vi "api_token.read.vi"(8 "error in":errorcluster, 11 "Nominal Client in":refnum<class "Nominal Client.lvclass">) -> (0 "error out":errorcluster, 2 "API Token":string, 3 "Nominal Client out":refnum<class "Nominal Client.lvclass">)   [LabVIEW 2020, in "Nominal Client.lvclass"]
uses:
  Nominal Client.lvclass
  Nominal Client.lvclass/Nominal Client.ctl
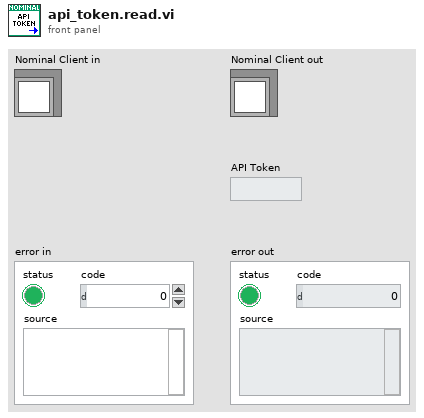
[diagram p1: front panel]
types:
  T1 = typedef "Nominal Client.lvclass/private_data.ctl" = cluster{"API Token":string, "REST Client":refnum<class "REST Client.lvclass">}
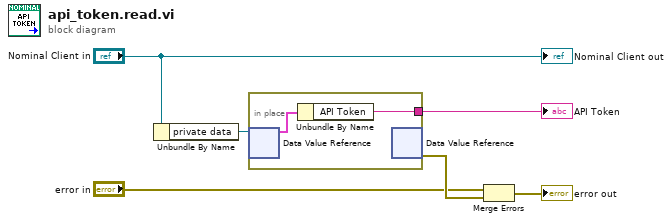
[diagram p0: block diagram]
diagram:
  n1 = Unbundle By Name("Nominal Client in") -> ("private data"=w6:refnum<data-value>)
  n2 = in-place {
    in-place-border: [w7] -> w5
    n3 = in-place-dvr #1(w6) -> (w8:T1)  [unwired: 1 out]
    n4 = Unbundle By Name(w8) -> ("API Token"=w7:string)
    n5 = in-place-dvr #1() -> (w3:errorcluster)  [unwired: 1 in, 1 out]
  }
  "API Token" <- w5
  n6 = Merge Errors("error in", w3) -> (→"error out":errorcluster)
  "Nominal Client out" <- "Nominal Client in"
